vi "DSF.Engine.Framework.Load Plugins.vi"(8 "error in (no error)":errorcluster, 11 "Framework in":refnum<class "DSF.Engine.Framework.lvclass">) -> (0 "error out":errorcluster, 2 "Plugins":refnum<class "DSF.Engine.Plugin.lvclass">[](array[class]), 3 "Framework out":refnum<class "DSF.Engine.Framework.lvclass">)   [LabVIEW 2017, in "DSF.Engine.lvlib" / "DSF.Engine.Framework.lvclass"]
uses:
  DSF.Engine.Framework.lvclass
  Plugin/DSF.Engine.Plugin.lvclass
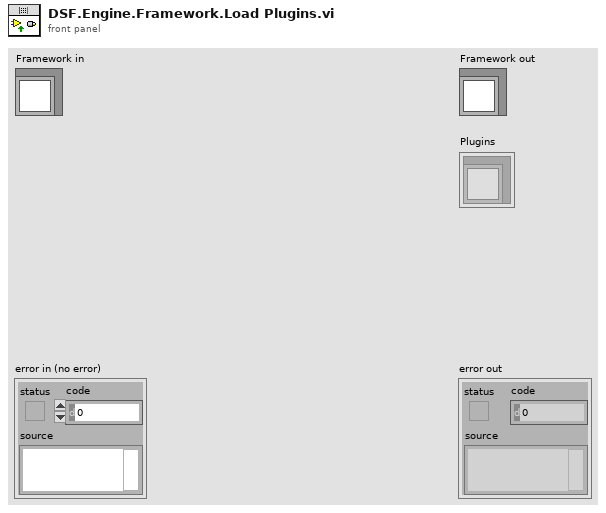
[diagram p1: front panel]
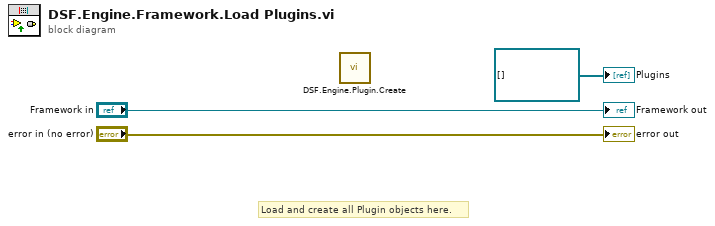
[diagram p0: block diagram]
diagram:
  # "Load and create all Plugin objects here."
  n1 = call "DSF.Engine.Plugin.Create.vi"() -> ()  [unwired: 10 in, 2 out]
  "error out" <- "error in (no error)"
  "Framework out" <- "Framework in"
  "Plugins" <- refnum<class "DSF.Engine.Plugin.lvclass">[] [] ("Transfers")
